vi "Get Time String.vi"() -> (2 "Time String":string)   [LabVIEW 2015]
uses:
  Clock Control Enum.ctl
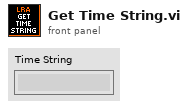
[diagram p1: front panel]
types:
  T1 = typedef "Clock Control Enum.ctl" = enum16{"Set", "Get", "Start", "Stop"}
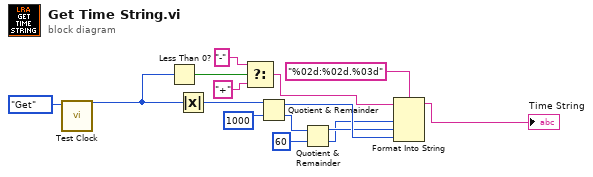
[diagram p0: block diagram]
diagram:
  n1 = call "Test Clock.vi"("Command"=Clock_Control_Enum."Get") -> ("Time"=w5:i32)  [unwired: 9 in, 1 out]
  n2 = Less Than 0?(x=w5) -> (x < 0?=w4:bool)
  n3 = Absolute Value(x=w5) -> (abs(x)=w6:i32)
  n4 = Select(t="-", s=w4, f="+") -> (s? t:f=w1:string)
  n5 = Quotient & Remainder(x=w6, y=1000) -> (x-y*floor(x/y)=w9:i32, floor(x/y)=w13:i32)
  n6 = Quotient & Remainder(x=w13, y=60) -> (x-y*floor(x/y)=w8:i32, floor(x/y)=w7:i32)
  n7 = Format Into String(format string="%02d:%02d.%03d", initial string=w1, w7, w8, w9) -> (resulting string=→"Time String":string)  [unwired: 1 in, 1 out]
